vi "CheckState.vi"(1 "™z²é î‘B":T1, 2 "Ïµ½y î‘B":refnum<vi>) -> (0 "ChkOK?":bool)   [LabVIEW 2012]
uses:
  SystemState.ctl
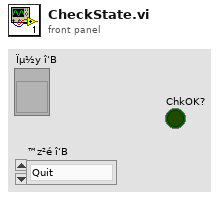
[diagram p1: front panel]
types:
  T1 = typedef "SystemState.ctl" = enum16{"Quit", "Error", "Stopping", "Starting", "Init", "Scan", "Menu", "ReadConf", "Idle"}
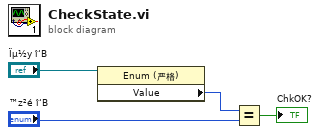
[diagram p0: block diagram]
diagram:
  n1 = property class="Enum (严格)"(reference="Ïµ½y î‘B") -> ("Value"=w2:T1)  [unwired: 1 in, 2 out]
  n2 = Equal?(x=w2, y="™z²é î‘B") -> (x = y?=→"ChkOK?":bool)
